vi "createState.vi"(8 "error in (no error)":errorcluster, 10 "stateValue":T1, 11 "IStateFactory in":refnum<class "IStateFactory.lvclass">) -> (0 "error out":errorcluster, 2 "state":refnum<class "State.lvclass">, 3 "IStateFactory out":refnum<class "IStateFactory.lvclass">)   [LabVIEW 2016, in "IStateFactory.lvclass"]
uses:
  IStateFactory.lvclass
  State/State.lvclass
  Typedefs/StateValue.ctl
  Typedefs/EXATypedefs.lvlib
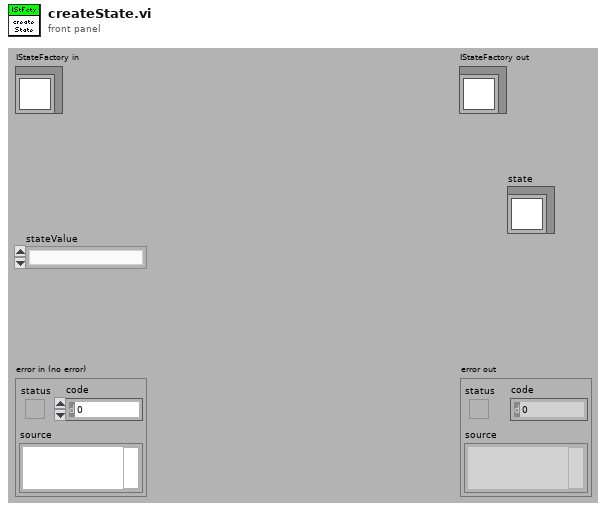
[diagram p1: front panel]
types:
  T1 = typedef "EXATypedefs.lvlib/StateValue.ctl" = enum16{"", " DisabledState", "EnabledState", "FaultState", "OfflineState", "StandbyState"}
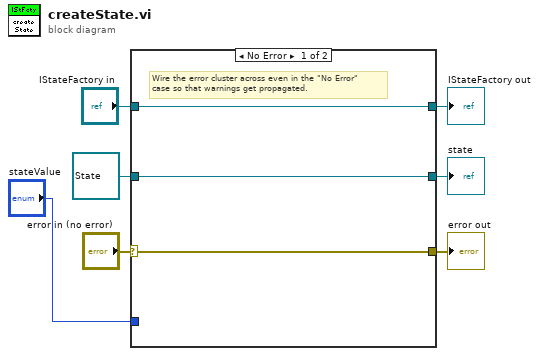
[diagram p0: block diagram]
diagram:
  n1 = case shown="No Error" "error in (no error)" {
    selector: "error in (no error)" -> [w9 w13]
    tunnel: [w9 w13] -> w6
    tunnel: [w10 w12] -> w4
    tunnel: "IStateFactory in" -> [w10 w12]
    tunnel: "stateValue" -> [_ _]
    tunnel: [w8 w11] -> w3
    tunnel: refnum<class "State.lvclass"> refnum ("State.lvclass") -> [w8 w11]
    frame No Error {
      # "Wire the error cluster across even in the \"No Error\"\ncase so that warnings get propagated."
    }
    frame Error {
    }
  }
  "error out" <- w6
  "IStateFactory out" <- w4
  "state" <- w3
